vi "SubVI_Files_to_epochs.vi"(6 "Ch_sel":i32[](array[numeric])=[0, 1, 1, 1, 0], 8 "error in (no error)":errorcluster, 9 "Restrict?":bool, 11 "folder names":string[](array[string])) -> (0 "error out":errorcluster, 1 "Number of Trials":i32, 2 "Rest Epochs":dbl[][](array[numeric]), 3 "Go Epochs":dbl[][](array[numeric]))   [LabVIEW 2020]
uses:
  <vilib>/Analysis/baseanly.llb/Mean (DBL).vi
  <vilib>/Analysis/NI_AALBase.lvlib
panel:
  out "Trial number":i32
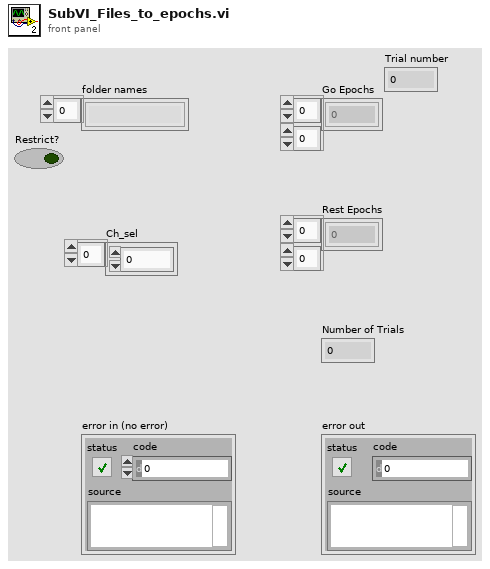
[diagram p1: front panel]
types:
  T1 = enum16{"open", "open or create", "create or replace", "create", "open (read-only)"}
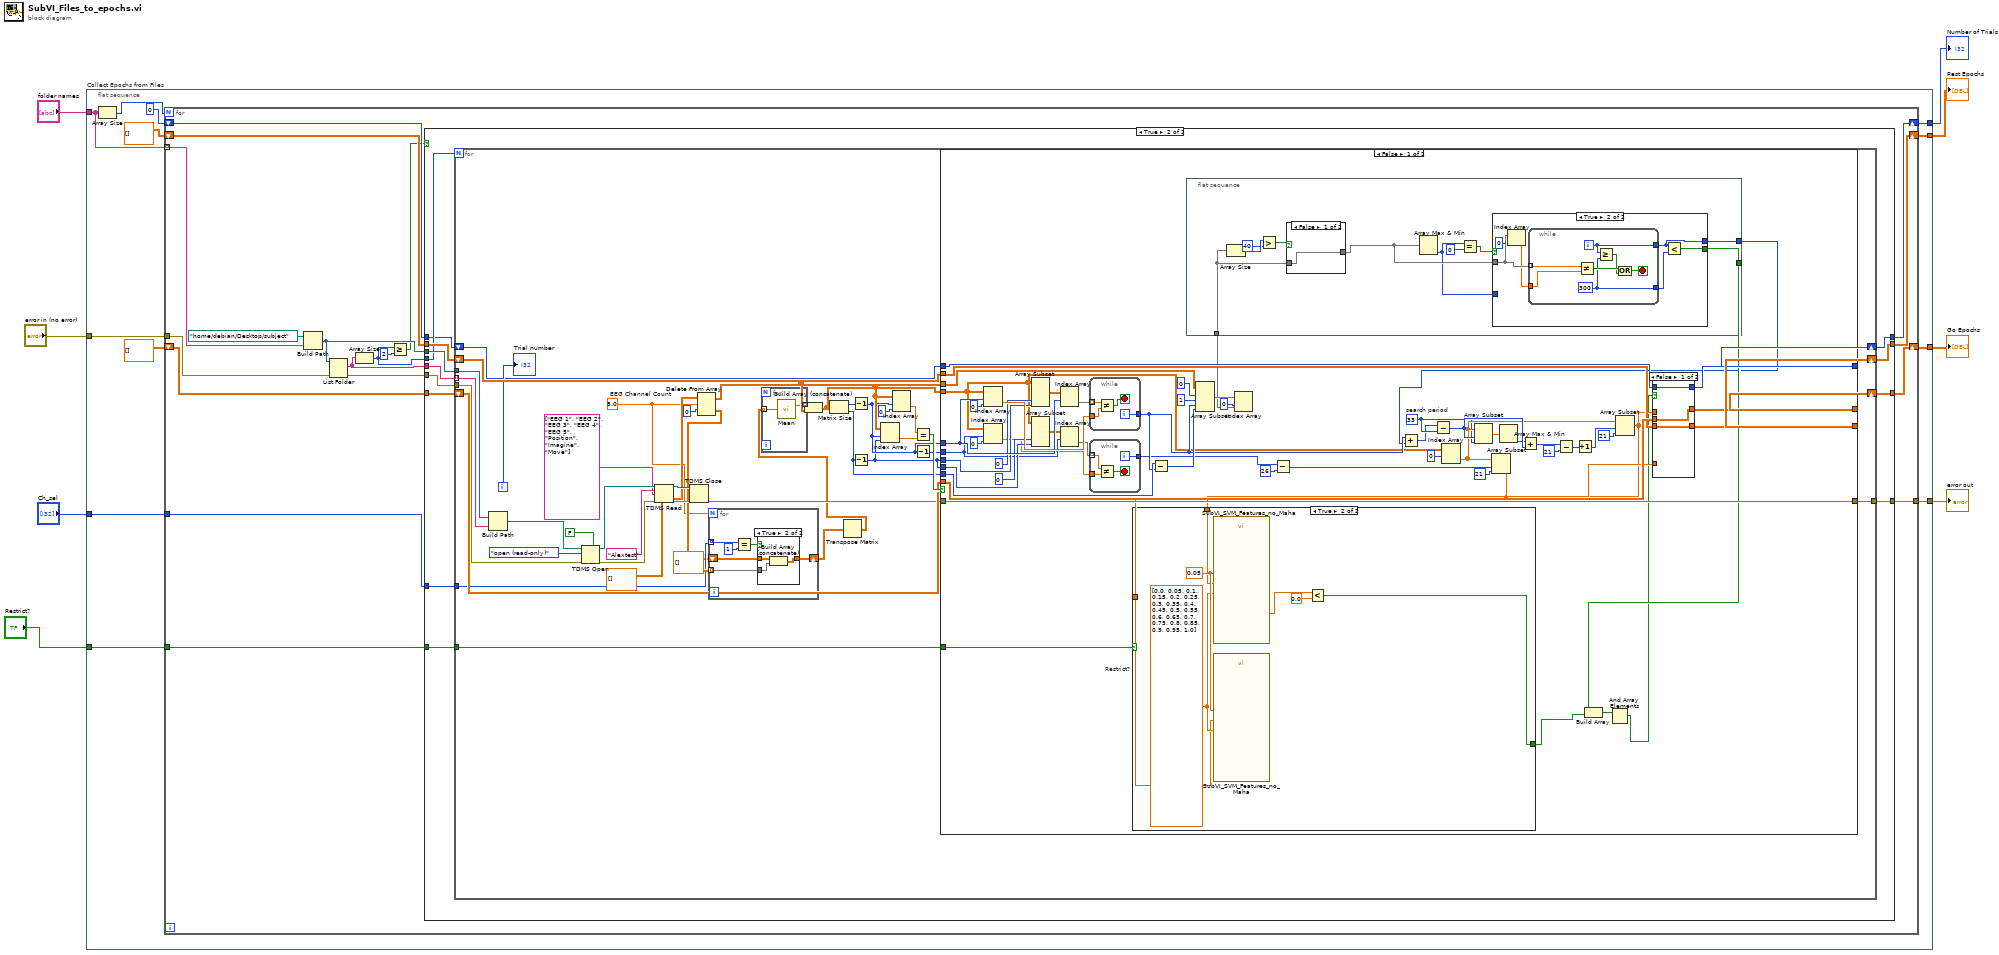
[diagram p0: block diagram]
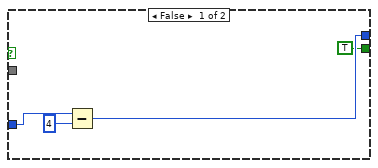
[diagram p4: hidden frame]
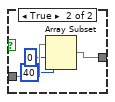
[diagram p5: hidden frame]
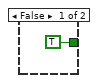
[diagram p6: hidden frame]
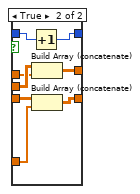
[diagram p7: hidden frame]
diagram:
  n1 = flat-sequence "Collect Epochs from Files" {
    tunnel: "folder names" -> [w19]
    tunnel: "error in (no error)" -> [w18]
    tunnel: [w15] -> w5
    tunnel: [w14] -> w6
    tunnel: [w13] -> w7
    tunnel: [w11] -> w8
    tunnel: "Restrict?" -> [w10]
    tunnel: "Ch_sel" -> [w9]
    frame #0 {
      n2 = Array Size(array=w19) -> (size(s)=w20:i32)
      n3 = for {
        N: w20 -> [_]
        tunnel: w19 -> [w38] mode=indexing
        tunnel: w18 -> [w37]
        tunnel: [w23] -> w13
        shift-right: [w32] -> w15
        shift-left: dbl[][] [] ("Data Buffer") -> [w33]
        shift-right: [w30] -> w14
        shift-left: dbl[][] [] ("Data Buffer") -> [w31]
        shift-right: [w28] -> w11
        shift-left: 0 -> [w29]
        tunnel: w10 -> [w22]
        tunnel: w9 -> [w21]
        n4 = Build Path(base path=path "/home/debian/Desktop/subject", name or relative path=w38) -> (appended path=w34:path)
        n5 = List Folder(path=w34, error in=w37) -> (filenames=w36:string[], error out=w24:errorcluster)  [unwired: 2 in, 2 out]
        n6 = Array Size(array=w36) -> (size(s)=w27:i32)
        n7 = Greater Or Equal?(x=w27, y=2) -> (x >= y?=w25:bool)
        n8 = case shown="True" w25 {
          tunnel: w36 -> [_ w55]
          tunnel: w34 -> [_ w54]
          tunnel: w33 -> [w41 w53]
          tunnel: [w41 w52] -> w32
          tunnel: w31 -> [w40 w51]
          tunnel: [w40 w50] -> w30
          tunnel: w29 -> [w42 w46]
          tunnel: w27 -> [_ w49]
          tunnel: [w42 w45] -> w28
          tunnel: w24 -> [w39 w48]
          tunnel: [w39 w47] -> w23
          tunnel: w22 -> [_ w44]
          tunnel: w21 -> [_ w43]
          frame False {
          }
          frame True {
            n9 = for {
              N: w49 -> [_]
              tunnel: w55 -> [w90] mode=indexing
              tunnel: w54 -> [w91]
              shift-right: [w81] -> w52
              shift-left: w53 -> [w82]
              shift-right: [w83] -> w50
              shift-left: w51 -> [w84]
              tunnel: w48 -> [w74]
              tunnel: [w69] -> w47
              shift-right: [w66] -> w45
              shift-left: w46 -> [w67]
              tunnel: w44 -> [w62]
              tunnel: w43 -> [w58]
              i -> [w68]
              w57 = 5.0  # EEG Channel Count
              n10 = Build Path(base path=w91, name or relative path=w90) -> (appended path=w89:path)
              n11 = TDMS Open(5:FALSE ("create index file? (T)"), 8:w74, 10:T1."open (read-only)" ("operation (0:open)"), 11:w89) -> (0:w95:errorcluster, 3:w93:refnum<k34>)  [unwired: 3 in]
              n12 = TDMS Read(0:w93, 5:"Alextest" ("group name in (Untitled)"), 7:string[] ["EEG 1", "EEG 2", "EEG 3", "EEG 4", "EEG 5", "Position", "Imagine", "Move"] ("channel name(s) in (Untitled)"), 11:w95, 12:dbl[][] [] ("Data Buffer")) -> (4:w92:refnum<k34>, 10:w78:dbl[][], 15:w94:errorcluster)  [unwired: 3 in, 3 out]
              n13 = TDMS Close(8:w94, 11:w92) -> (0:w70:errorcluster)  [unwired: 1 out]
              n14 = Delete From Array(array=w78, length=w57, index (row)=0) -> (deleted portion=w61:dbl[][], array with subset deleted=w72:dbl[][])  [unwired: 1 in]
              n15 = for {
                N: w57 -> [_]
                tunnel: w61 -> [w101] mode=indexing
                tunnel: w58 -> [w104] mode=indexing
                shift-right: [w100] -> w60
                shift-left: dbl[][] [] -> [w99]
                n16 = Equal?(x=w104, y=1) -> (x = y?=w102:bool)
                n17 = case shown="True" w102 {
                  tunnel: w101 -> [_ w108]
                  tunnel: [w105 w107] -> w100
                  tunnel: w99 -> [w105 w106]
                  frame False {
                  }
                  frame True {
                    n18 = Build Array (concatenate)(w106, w108) -> (w107:dbl[][])
                  }
                }
              }
              n19 = Transpose Matrix(1:w60) -> (0:w59:dbl[][])
              n20 = for {
                tunnel: w59 -> [w110] mode=indexing
                tunnel: [w109] -> w76 mode=indexing
                n21 = call-poly <vilib>:"Mean.vi"("X"=w110) -> ("mean"=w109:dbl)  [unwired: 1 out]
              }
              n22 = Build Array (concatenate)(w76, w72) -> (w75:dbl[][])
              n23 = Matrix Size(0:w75) -> (1:w79:i32, 2:w71:i32)
              n24 = Decrement(x=w79) -> (x-1=w65:i32)
              n25 = Decrement(x=w71) -> (x-1=w63:i32)
              n26 = Index Array(array=w75, index (row)=w65, index (col)=w63) -> (element=w86:dbl)
              n27 = Index Array(array=w75, index (row)=w65, index (col)=0 ("disabled index (col)")) -> (element=w87:dbl)
              n28 = Equal?(x=w87, y=w86) -> (x = y?=w85:bool)
              n29 = Decrement(x=w65) -> (x-1=w64:i32)
              n30 = case shown="False" w85 {
                tunnel: w84 -> [w150 w228]
                tunnel: [w149 w228] -> w83
                tunnel: w82 -> [w152 w227]
                tunnel: [w151 w227] -> w81
                tunnel: w75 -> [w130 _]
                tunnel: w65 -> [w147 _]
                tunnel: w63 -> [w145 _]
                tunnel: w72 -> [w142 _]
                tunnel: w71 -> [w141 _]
                tunnel: w70 -> [w134 w226]
                tunnel: [w134 w226] -> w69
                tunnel: w67 -> [w132 w225]
                tunnel: [w131 w225] -> w66
                tunnel: w64 -> [w125 _]
                tunnel: w63 -> [w126 _]
                tunnel: w62 -> [w117 _]
                frame False {
                  w143 = 33  # search period
                  n31 = Index Array(array=w130, index (row)=w147, index (col)=0 ("disabled index (col)")) -> (element=w163:dbl)
                  n32 = Index Array(array=w130, index (row)=w125, index (col)=0 ("disabled index (col)")) -> (element=w123:dbl)
                  n33 = Array Subset(array=w130, index (col)=0 ("index"), length (col)=w145) -> (w148:dbl[][])  [unwired: 2 in]
                  n34 = Array Subset(array=w130, index (col)=0 ("index"), length (col)=w126) -> (w129:dbl[][])  [unwired: 2 in]
                  n35 = Index Array(array=w148, index (row)=w147) -> (element=w165:dbl[])  [unwired: 1 in]
                  n36 = Index Array(array=w129, index (row)=w125) -> (element=w124:dbl[])  [unwired: 1 in]
                  n37 = while {
                    tunnel: w165 -> [w222] mode=indexing
                    tunnel: w163 -> [w223]
                    tunnel: [w221] -> w133
                    i -> [w221]
                    stop <- w224 stop-if-true
                    n38 = Not Equal?(x=w222, y=w223) -> (x != y?=w224:bool)
                  }
                  n39 = while {
                    tunnel: w124 -> [w207] mode=indexing
                    tunnel: w123 -> [w208]
                    tunnel: [w206] -> w122
                    i -> [w206]
                    stop <- w209 stop-if-true
                    n40 = Not Equal?(x=w207, y=w208) -> (x != y?=w209:bool)
                  }
                  n41 = Subtract(x=w141, y=w133) -> (x-y=w140:i32)
                  n42 = flat-sequence {
                    tunnel: w116 -> [w172]
                    tunnel: [w168] -> w115
                    tunnel: [w166] -> w111
                    frame #0 {
                      n43 = Array Size(array=w172) -> (size(s)=w175:i32)
                      n44 = Greater?(x=w175, y=40) -> (0:w173:bool)
                      n45 = case shown="False" w173 {
                        tunnel: w172 -> [w193 w197]
                        tunnel: [w193 w194] -> w169
                        frame False {
                        }
                        frame True {
                          n46 = Array Subset(array=w197, index=0, length=40) -> (w194:dbl[])
                        }
                      }
                      n47 = Array Max & Min(array=w169) -> (min index (indices)=w167:i32)  [unwired: 3 out]
                      n48 = Equal?(x=w167, y=0) -> (x = y?=w170:bool)
                      n49 = case shown="True" w170 {
                        tunnel: w169 -> [_ w185]
                        tunnel: [TRUE w181] -> w168
                        tunnel: [w177 w180] -> w166
                        tunnel: w167 -> [w179 _]
                        frame False {
                          n50 = Subtract(x=w179, y=4) -> (x-y=w177:i32)
                        }
                        frame True {
                          n51 = Index Array(array=w185, index=0) -> (element=w183:dbl)
                          n52 = while {
                            tunnel: w185 -> [w192] mode=indexing
                            tunnel: [w189] -> w180
                            tunnel: [w187] -> w182
                            tunnel: w183 -> [w186]
                            i -> [w189]
                            stop <- w188 stop-if-true
                            w187 = 300 ("y")
                            n53 = Not Equal?(x=w192, y=w186) -> (x != y?=w191:bool)
                            n54 = Greater Or Equal?(x=w189, y=w187) -> (x >= y?=w190:bool)
                            n55 = Or(x=w191, y=w190) -> (x .or. y?=w188:bool)
                          }
                          n56 = Less?(x=w180, y=w182) -> (x < y?=w181:bool)
                        }
                      }
                    }
                  }
                  n57 = Array Subset(array=w142, index (row)=0 ("index"), length (row)=1 ("length"), index (col)=w133, length (col)=w140) -> (w138:dbl[][])
                  n58 = Index Array(array=w138, index (row)=0) -> (element=w116:dbl[])  [unwired: 1 in]
                  n59 = Subtract(x=w122, y=26) -> (x-y=w120:i32)
                  n60 = Add(x=w133, y=w111) -> (x+y=w139:i32)
                  n61 = Subtract(x=w139, y=w143) -> (x-y=w160:i32)
                  n62 = Index Array(array=w130, index (row)=0) -> (element=w154:dbl[])  [unwired: 1 in]
                  n63 = Array Subset(array=w154, index=w160, length=w143) -> (w161:dbl[])
                  n64 = Array Subset(array=w154, index=w120, length=21) -> (w119:dbl[])
                  n65 = Array Max & Min(array=w161) -> (min index (indices)=w159:i32)  [unwired: 3 out]
                  n66 = Add(x=w159, y=w160) -> (x+y=w158:i32)
                  n67 = Subtract(x=w158, y=21) -> (x-y=w156:i32)
                  n68 = Increment(x=w156) -> (x+1=w144:i32)
                  n69 = Array Subset(array=w154, index=w144, length=21) -> (w118:dbl[])
                  n70 = case "Restrict?" shown="True" w117 {
                    tunnel: w119 -> [_ w203]
                    tunnel: w118 -> [_ w202]
                    tunnel: [TRUE w199] -> w112
                    frame False {
                    }
                    frame True {
                      w205 = 0.05 ("dt")
                      w204 = dbl[] [0.0, 0.05, 0.1, 0.15, 0.2, 0.25, 0.3, 0.35, 0.4, 0.45, 0.5, 0.55, 0.6, 0.65, 0.7, 0.75, 0.8, 0.85, 0.9, 0.95, 1.0] ("Sliding_window")
                      n71 = call "SubVI_SVM_Features_no_Maha.vi"("dt"=w205, "window_time"=w204, "Sliding_window"=w202) -> ("min value"=w201:dbl)  [unwired: 5 in, 3 out]
                      n72 = call "SubVI_SVM_Features_no_Maha.vi"("dt"=w205, "window_time"=w204, "Sliding_window"=w203) -> ()  [unwired: 5 in, 4 out]
                      n73 = Less?(x=w201, y=0.0) -> (x < y?=w199:bool)
                    }
                  }
                  n74 = Build Array(w115, w112) -> (w114:bool[])
                  n75 = And Array Elements(Boolean array=w114) -> (logical AND=w113:bool)
                  n76 = case shown="False" w113 {
                    tunnel: w152 -> [w212 w220]
                    tunnel: w118 -> [_ w219]
                    tunnel: [w212 w218] -> w151
                    tunnel: w150 -> [w211 w217]
                    tunnel: w119 -> [_ w216]
                    tunnel: [w211 w215] -> w149
                    tunnel: w132 -> [w210 w214]
                    tunnel: [w210 w213] -> w131
                    frame False {
                    }
                    frame True {
                      n77 = Increment(x=w214) -> (x+1=w213:i32)
                      n78 = Build Array (concatenate)(w220, w219) -> (w218:dbl[][])
                      n79 = Build Array (concatenate)(w217, w216) -> (w215:dbl[][])
                    }
                  }
                }
                frame True {
                }
              }
              "Trial number" <- w68
            }
          }
        }
      }
    }
  }
  "Number of Trials" <- w8
  "error out" <- w7
  "Rest Epochs" <- w6
  "Go Epochs" <- w5
